vi "PostProcess.vi"(8 "error in (no error)":errorcluster, 10 "Variant in":variant, 11 "ONNX EfficientNet Class in":refnum<class "ONNX EfficientNet Class.lvclass">) -> (0 "error out":errorcluster, 2 "Variant out":variant, 3 "ONNX EfficientNet Class out":refnum<class "ONNX EfficientNet Class.lvclass">)   [LabVIEW 2017, in "ONNX EfficientNet Class Library.lvlib" / "ONNX EfficientNet Class.lvclass"]
uses:
  ONNX EfficientNet Class.lvclass
  ONNX EfficientNet Class.lvclass/ONNX EfficientNet Class.ctl
panel:
  out "result":cluster{"conf":sgl, "class":string}[](array[cluster])
  out "conf":sgl[](array[numeric])
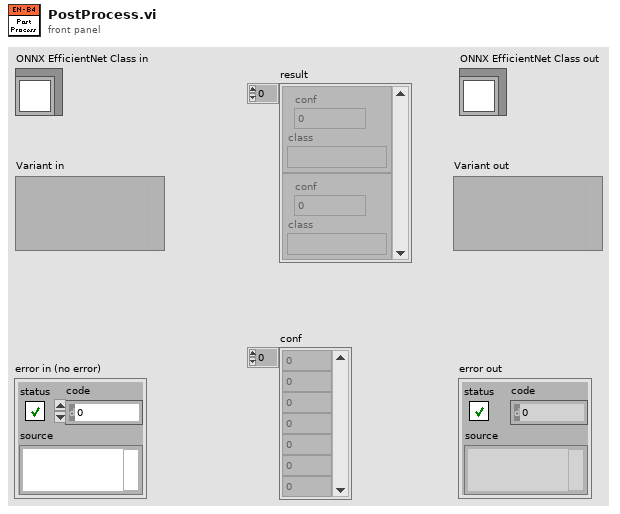
[diagram p1: front panel]
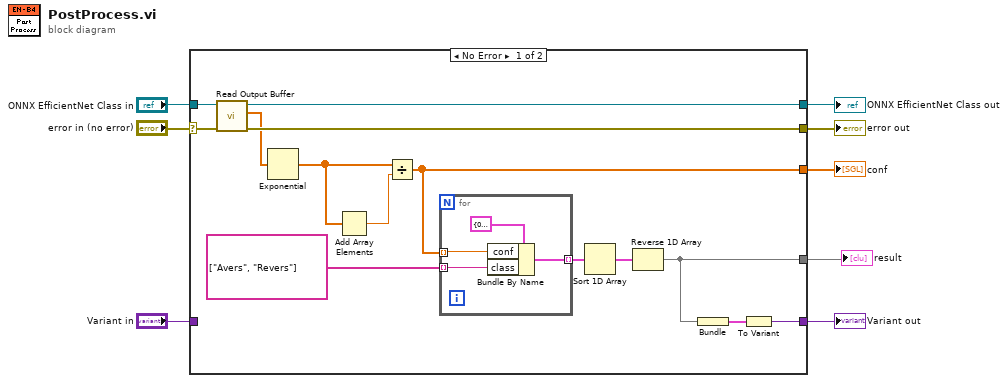
[diagram p0: block diagram]
diagram:
  n1 = case shown="No Error" "error in (no error)" {
    selector: "error in (no error)" -> [w18 w27]
    tunnel: "Variant in" -> [_ w28]
    tunnel: "ONNX EfficientNet Class in" -> [w22 w29]
    tunnel: [w21 w29] -> w4
    tunnel: [w19 w28] -> w5
    tunnel: [w20 w27] -> w3
    tunnel: [w11 _] -> w2
    tunnel: [w10 _] -> w1
    frame No Error {
      n2 = call-dynamic "Read Output Buffer.vi"("error in (no error)"=w18, "ONNX Class in"=w22) -> ("error out"=w20:errorcluster, "Output Buffer"=w12:sgl[], "ONNX Class out"=w21:refnum<class "ONNX EfficientNet Class.lvclass">)  [unwired: 7 in]
      n3 = Exponential(1:w12) -> (0:w14:sgl[])
      n4 = Add Array Elements(numeric array=w14) -> (sum=w15:sgl)
      n5 = Divide(x=w14, y=w15) -> (x/y=w11:sgl[])
      n6 = for {
        tunnel: w11 -> [w26] mode=indexing
        tunnel: string[] ["Avers", "Revers"] -> [w24] mode=indexing
        tunnel: [w23] -> w16 mode=indexing
        n7 = Bundle By Name(cluster=cluster{"conf":sgl, "class":string} {"conf"=0.0, "class"=""} ("input cluster"), "conf"=w26, "class"=w24) -> (w23:cluster{"conf":sgl, "class":string})
      }
      n8 = Sort 1D Array(array=w16) -> (sorted array=w17:cluster{"conf":sgl, "class":string}[])
      n9 = Reverse 1D Array(array=w17) -> (reversed array=w10:cluster{"conf":sgl, "class":string}[])
      n10 = Bundle(w10) -> (w9:cluster{cluster{"conf":sgl, "class":string}[]})  [unwired: 1 in]
      n11 = To Variant(anything=w9) -> (Variant=w19:variant)
    }
    frame Error {
    }
  }
  "error out" <- w3
  "ONNX EfficientNet Class out" <- w4
  "Variant out" <- w5
  "conf" <- w2
  "result" <- w1
